vi "Write Results Queue.vi"(8 "error in (no error)":errorcluster, 10 "Results Queue":refnum<queue>, 11 "Launch Measurement and Wait for Result in":refnum<class "Launch Measurement and Wait for Result.lvclass">) -> (0 "error out":errorcluster, 3 "Launch Measurement and Wait for Result out":refnum<class "Launch Measurement and Wait for Result.lvclass">)   [LabVIEW 2026, in "Controller API.lvlib" / "Launch Measurement and Wait for Result.lvclass"]
uses:
  Launch Measurement and Wait for Result.lvclass
  Launch Measurement and Wait for Result.lvclass/Launch Measurement and Wait for Result.ctl
  framework/Results/Results.lvclass
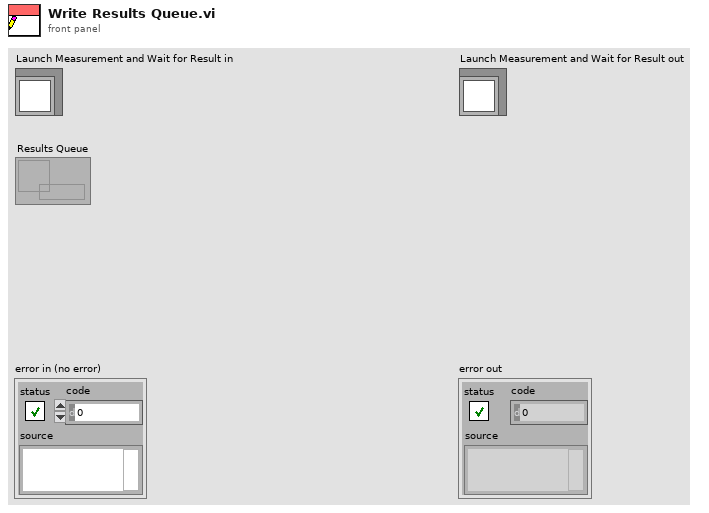
[diagram p1: front panel]
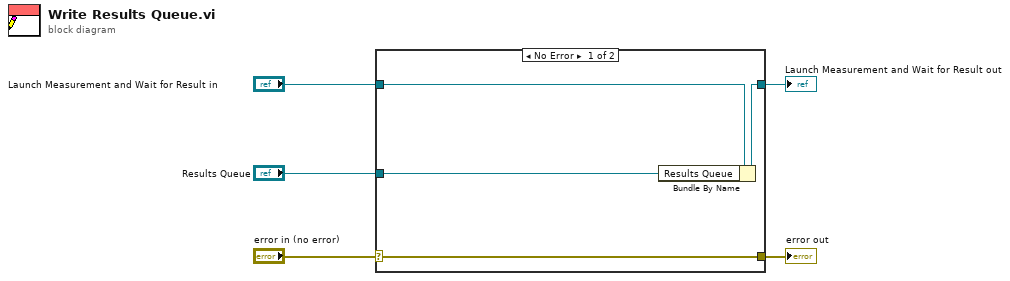
[diagram p0: block diagram]
diagram:
  n1 = case shown="No Error" "error in (no error)" {
    selector: "error in (no error)" -> [w9 w10]
    tunnel: [w9 w10] -> w4
    tunnel: [w7 w11] -> w2
    tunnel: "Launch Measurement and Wait for Result in" -> [w8 w11]
    tunnel: "Results Queue" -> [w6 _]
    frame No Error {
      n2 = Bundle By Name(cluster=w8, "Results Queue"=w6) -> (w7:refnum<class "Launch Measurement and Wait for Result.lvclass">)
    }
    frame Error {
    }
  }
  "error out" <- w4
  "Launch Measurement and Wait for Result out" <- w2
